vi "NI-DCPower Source DC Current.vi"() -> ()   [LabVIEW 2021, in "DCCurrent.lvlib"]
doc: "Demonstrates how to use the DC Current Output Function to force an output current. This example initializes a session, configures the Output Function, Sense, Autorange, Current Level and Voltage Limit, initiates generation, waits for a specified delay, and measures the voltage and current output. This example uses Single Point source mode."
uses:
  DCCurrent.lvlib
  controls/Test.ctl
  controls/Measurements.ctl
panel:
  out "Measurements":T1
  in  "error in":errorcluster
  out "error out":errorcluster
  in  "Source Delay (Sec)":dbl=0.1 format="%.3p"
  in  "Voltage Limit Range":dbl=6.0 format="%.5p"
  in  "Current Level Range":dbl=0.01 format="%.3p"
  in  "Voltage Limit":dbl=2.0 format="%.5p"
  in  "Current Level":T2=0.01 format="%.3p"
  in  "Load SMU Channel":string="0"
  in  "Load SMU":refnum<k15>="Dev1"
  # "Overview: Demonstrates how to use the DC Current Output Function to force an output current.  \nThis example initializes a session; configures the Output Function, Current Level and Voltage Limit; \ninitiates generation; waits for a specified delay; and measures the voltage and current output.  \nRequirements: NI-DCPower\nInstructions:\n1. Select the appropriate device in the Resource Name control.\n2. Configure the parameters of the DC Current signal you'd like to output.\n3. Run the VI."
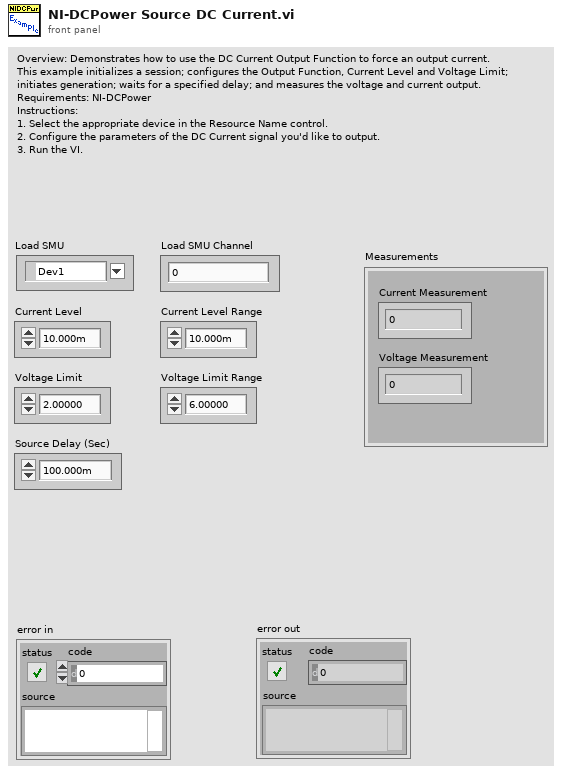
[diagram p1: front panel]
types:
  T1 = typedef "Measurements.ctl" = cluster{"Current Measurement":dbl, "Voltage Measurement":dbl}
  T2 = typedef "Test.ctl" = dbl
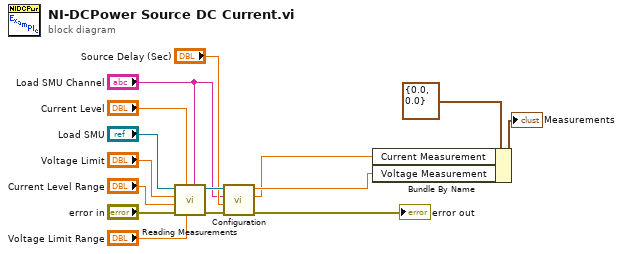
[diagram p0: block diagram]
diagram:
  n1 = call "Reading Measurements.vi"("Load SMU Channel"="Load SMU Channel", "Voltage Limit Range"="Voltage Limit Range", "Current Level"="Current Level", "error in (no error)"="error in", "Current Level Range"="Current Level Range", "Voltage Limit"="Voltage Limit", "IVI Refnum in"="Load SMU") -> ("error out"=w9:errorcluster, "IVI Refnum out"=w10:refnum<k15>)  [unwired: 3 in]
  n2 = call "Configuration.vi"("error in (no error)"=w9, "Source Delay (Sec)"="Source Delay (Sec)", "Load SMU Channel"="Load SMU Channel", "IVI Refnum in"=w10) -> ("error out"=→"error out":errorcluster, "Current Measurement"=w1:dbl, "Voltage Measurement"=w2:dbl)  [unwired: 5 in]
  n3 = Bundle By Name(cluster=T1 {"Current Measurement"=0.0, "Voltage Measurement"=0.0} ("Measurements"), "Current Measurement"=w1, "Voltage Measurement"=w2) -> (→"Measurements":T1)
